vi "Fetch a Table from VAC DB_140603.vi"() -> ()   [LabVIEW 2011]
doc: "This example opens a connection to a database specified by the Connection string (replace the DNS name with your database) and retrieves all the rows and columns from the table \"Table1\" (replace the SQL string with your own SQL query)."
panel:
  in  "Command Text 2":string="select * from bkbranch;"
  in  "ConnectionString 2":string="Provider=sqloledb;Server=140.93.100.252;User ID=vac103;Password=vac@123456;Database=scholarship;"
  out "Command Text":string="SHOW TABLES LIMIT 10;"
  out "ConnectionString":string="Provider=sqloledb;Server=140.93.100.252;User ID=vac103;Password=vac@123456;Database=HR_VAC;"
  out "error out":errorcluster
  out "SQL Results":string[][](table)
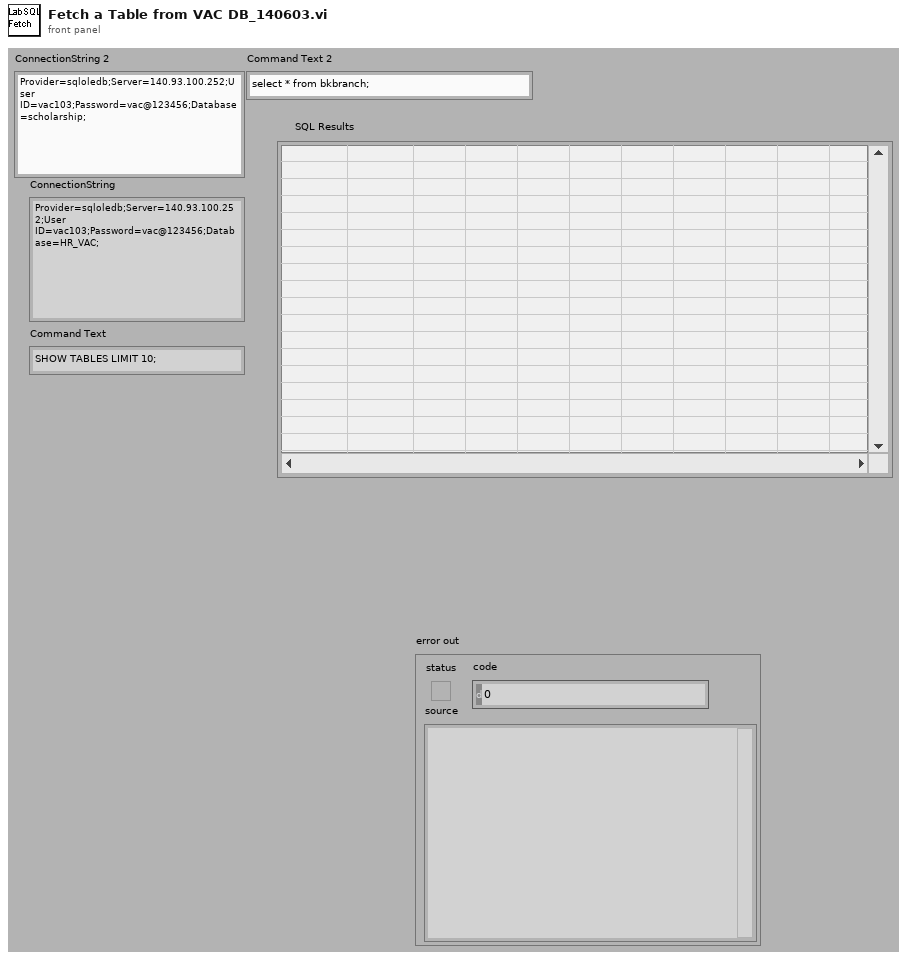
[diagram p1: front panel]
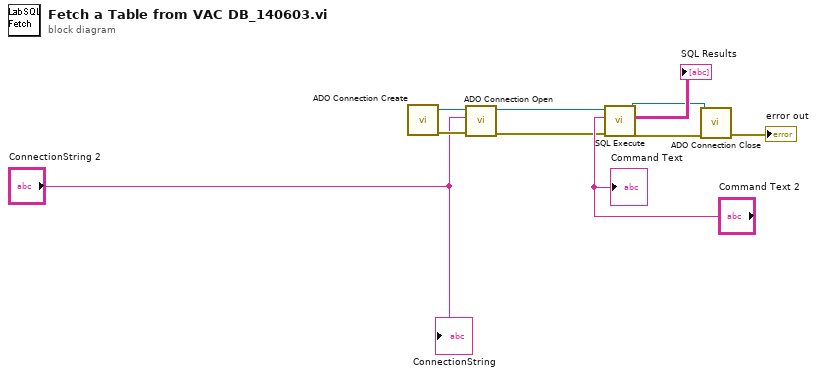
[diagram p0: block diagram]
diagram:
  n1 = call "ADO Connection Create.vi"() -> ("error out"=w9:errorcluster, "ADODB._Connection Out"=w10:refnum<k7>)  [unwired: 10 in]
  n2 = call "ADO Connection Open.vi"("error in (no error)"=w9, "ConnectionString"="ConnectionString 2", "ADODB._Connection In"=w10) -> ("error out"=w5:errorcluster, "ADODB._Connection Out"=w7:refnum<k7>)  [unwired: 7 in]
  n3 = call "SQL Execute.vi"("error in (no error)"=w5, "Command Text"="Command Text 2", "ADODB._Connection In"=w7) -> ("error out"=w3:errorcluster, "Data"=→"SQL Results":string[][], "ADODB._Connection Out"=w2:refnum<k7>)  [unwired: 5 in, 1 out]
  n4 = call "ADO Connection Close.vi"("error in (no error)"=w3, "ADODB._Connection In"=w2) -> ("error out"=→"error out":errorcluster)  [unwired: 8 in, 1 out]
  "ConnectionString" <- "ConnectionString 2"
  "Command Text" <- "Command Text 2"
